vi "MALT Set Several.vi"(7 "MALT CardType":T1=enum."MALT160T", 8 "error in":errorcluster, 9 "State":bool, 10 "State Map":u8[](array[numeric]) format="%02x", 11 "Address":i32) -> (0 "error out":errorcluster)   [LabVIEW 2018, in "AltonTech MALT200817.lvlib"]
uses:
  AltonTech MALT200817.lvlib
  Types/MALT CardTypes.ctl
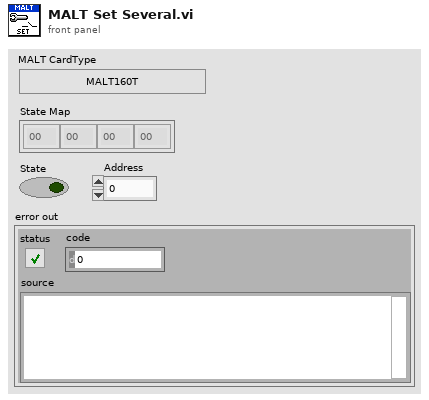
[diagram p1: front panel]
types:
  T1 = typedef "AltonTech MALT200817.lvlib/MALT CardTypes.ctl" = enum32{"-", "YAV90832", "YAV904X8", "MALT132", "YAV91616", "YAV90PIN", "YAV90096", "YAV90HVT", "YAV90CLR", "YAV90128", "YAV90PNE", "YAVCANCON", "YAV91775", "YAV90XXX", "YAV90MMU", "H730050", "H710060", "H710061", "YAV90304", "MMI", "YAV90060", "MALT160T", "YAV90059", "Not Defined"}
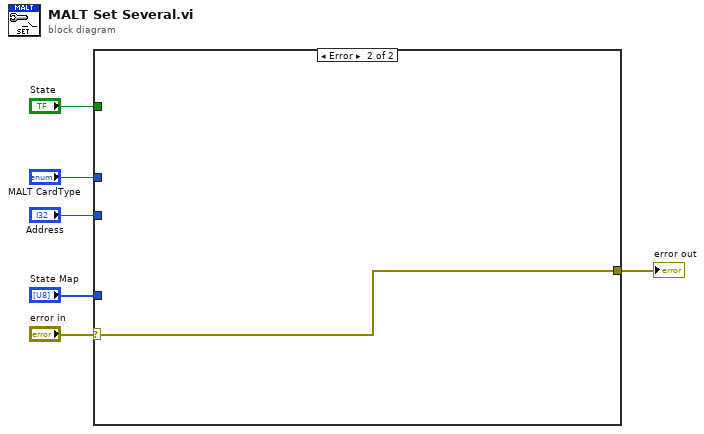
[diagram p0: block diagram]
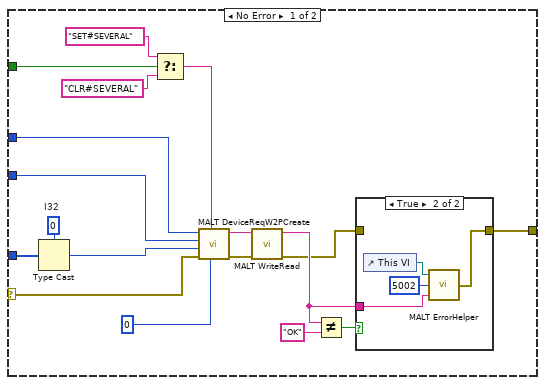
[diagram p2: hidden frame]
diagram:
  n1 = case shown="Error" "error in" {
    selector: "error in" -> [w7 w30]
    tunnel: "Address" -> [w22 _]
    tunnel: "MALT CardType" -> [w21 _]
    tunnel: [w17 w30] -> w4
    tunnel: "State" -> [w12 _]
    tunnel: "State Map" -> [w11 _]
    frame No Error {
      w10 = 0  # I32
      n2 = Type Cast(type=w10, x=w11) -> (*(type *) &x=w9:i32)
      n3 = Select(t="SET#SEVERAL" ("cmd"), s=w12, f="CLR#SEVERAL" ("cmd")) -> (s? t:f=w15:string)
      n4 = call "MALT DeviceReqW2PCreate.vi"("Param2"=0, "Cmd"=w15, "error in"=w7, "Param1"=w9, "Address"=w22, "CardType"=w21) -> ("error out"=w23:errorcluster, "Request"=w24:string)  [unwired: 4 in]
      n5 = call "MALT WriteRead.vi"("error in"=w23, "Request"=w24) -> ("error out"=w16:errorcluster, "Response"=w18:string)  [unwired: 8 in]
      n6 = Not Equal?(x=w18, y="OK") -> (x != y?=w19:bool)
      n7 = case shown="True" w19 {
        tunnel: w18 -> [_ w27]
        tunnel: [w25 w26] -> w17
        tunnel: w16 -> [w25 _]
        frame False {
        }
        frame True {
          n8 = control-ref of="This VI"() -> (w29:refnum<vi>)
          n9 = call "MALT ErrorHelper.vi"("Message"=w27, "Code"=5002, "This VI"=w29) -> ("error out"=w26:errorcluster)
        }
      }
    }
    frame Error {
    }
  }
  "error out" <- w4
